vi "Simulate XY Sensor Measurements.vi"(8 "Dynamical System Matrices":T3, 10 "Sensors":T2[](array[typedef]), 11 "Current State":T1) -> (3 "Observations":T1)   [LabVIEW 2020]
uses:
  ctl/Dynamical System Matrices.ctl
  <vilib>/Analysis/Matrix/Datatypes/RealMatrix.ctl
  ctl/XY (Position-Velocity) Sensor Instance.ctl
  <vilib>/Analysis/baseanly.llb/Real A x B.vi
  <vilib>/Analysis/Matrix/Numeric/Conversions/Array To Matrix - RA.vi
  <vilib>/Analysis/Matrix/Numeric/Add/Add - RM,RM.vi
  <vilib>/Analysis/NI_AALBase.lvlib
  <vilib>/Analysis/Matrix/NI_Matrix.lvlib
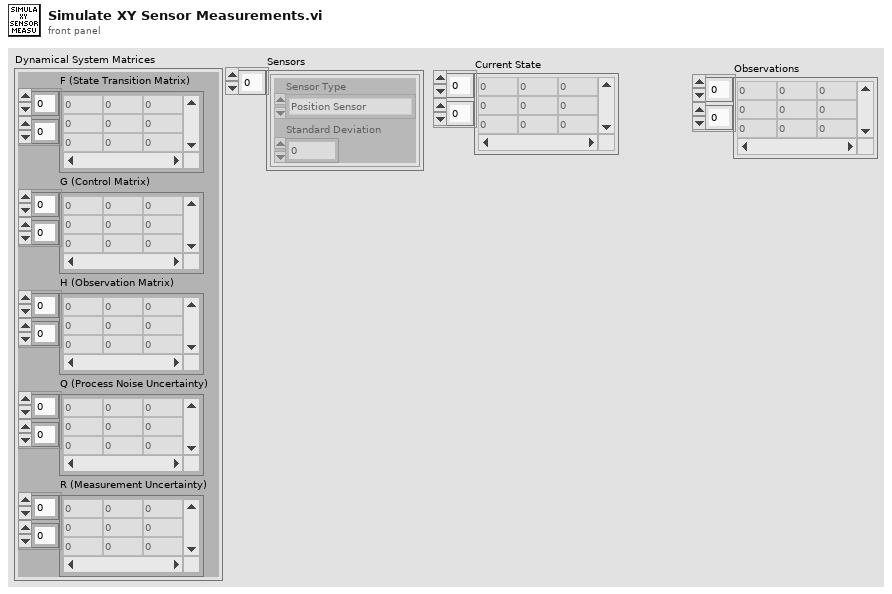
[diagram p1: front panel]
types:
  T1 = typedef "NI_Matrix.lvlib/RealMatrix.ctl" = dbl[][]
  T2 = typedef "XY (Position-Velocity) Sensor Instance.ctl" = cluster{"Sensor Type":enum16{"Position Sensor", "Velocity Sensor"}, "Standard Deviation":dbl}
  T3 = typedef "Dynamical System Matrices.ctl" = cluster{"F (State Transition Matrix)":T1, "G (Control Matrix)":T1, "H (Observation Matrix)":T1, "Q (Process Noise Uncertainty)":T1, "R (Measurement Uncertainty)":T1}
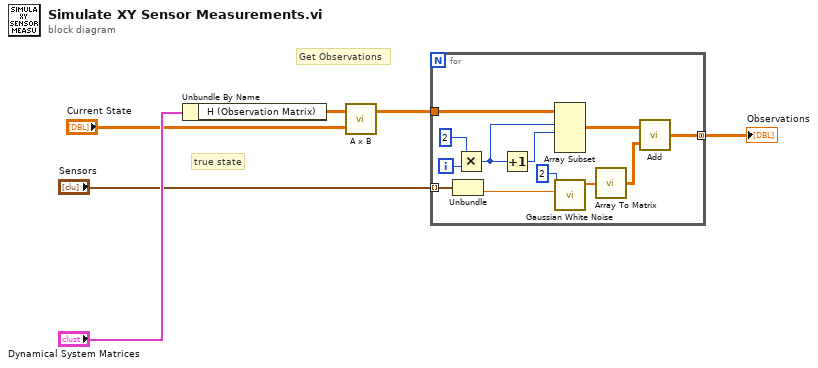
[diagram p0: block diagram]
diagram:
  # "Get Observations"
  # "true state"
  n1 = Unbundle By Name("Dynamical System Matrices") -> ("H (Observation Matrix)"=w5:T1)
  n2 = call-poly <vilib>:"A x B.vi"("B"="Current State", "A"=w5) -> ("A x B"=w6:T1)  [unwired: 1 out]
  n3 = for {
    tunnel: "Sensors" -> [w18] mode=indexing
    tunnel: w6 -> [w17]
    tunnel: [w9] -> w1 mode=concatenating
    i -> [w16]
    n4 = Unbundle(w18) -> ("Standard Deviation"=w13:dbl)  [unwired: 1 out]
    n5 = Multiply(x=2, y=w16) -> (x*y=w8:i32)
    n6 = Increment(x=w8) -> (x+1=w7:i32)
    n7 = Array Subset(array=w17, index (row)=w8, length (row)=w7) -> (w11:T1)  [unwired: 2 in]
    n8 = call <vilib>:"Gaussian White Noise.vi"("standard deviation"=w13, "samples"=2) -> ("Gaussian noise pattern"=w12:dbl[])  [unwired: 8 in, 1 out]
    n9 = call-poly <vilib>:"Array To Matrix.vi"("Real 1D Array"=w12) -> ("Real Matrix (Column Vector)"=w10:T1)
    n10 = call-poly <vilib>:"Add.vi"("Real Matrix B"=w10, "Real Matrix A"=w11) -> ("A + B"=w9:T1)
  }
  "Observations" <- w1
